vi "Inv_Mpemba1_flat potential_Host.vi"() -> ()   [LabVIEW 2019]
uses:
  <vilib>/rvi/interface/nirviMethod/nirviMethod.xnode
  <vilib>/rvi/errors/niLvFpgaMergeErrorWithErrorCode.vi
  <vilib>/rvi/interface/nirviReadWriteControl/nirviReadWriteControl.xnode
  <vilib>/rvi/interface/Simulation/niFpgaSimulationCallBeginRW.vi
  <vilib>/rvi/errors/niLvFpgaAdjustHostInterfaceError.vi
  <vilib>/Utility/file.llb/Write Delimited Spreadsheet (DBL).vi
  <vilib>/Analysis/NI_AALBase.lvlib
  <vilib>/Analysis/baseanly.llb/Mean (DBL).vi
  <vilib>/FPGAPlugInAG/Dynamic/niLvFpga_Reset_Dynamic.vi
  <vilib>/FPGAPlugInAG/Dynamic/niLvFpga_Run_Dynamic.vi
  <vilib>/rvi/interface/nirviCloseFPGA/nirviCloseFPGA.xnode
  <vilib>/rvi/interface/nirviOpenFPGA/nirviOpenFPGA.xnode
  <vilib>/FPGAPlugInAG/Dynamic/niLvFpga_ConfigureFifo_Dynamic.vi
  <vilib>/FPGAPlugInAG/Dynamic/niLvFpga_StartFifo_Dynamic.vi
  <vilib>/FPGAPlugInAG/Dynamic/niLvFpga_ReadFifo_Dynamic.vi
  <vilib>/FPGAPlugInAG/Dynamic/niLvFpga_StopFifo_Dynamic.vi
  <vilib>/FPGAPlugInAG/Dynamic/niLvFpga_Close_Dynamic.vi
panel:
  in  "Fiting Control":enum32{"Fitting Control", "Fitting Errors"}(tab)
  in  "initial\nparameters":dbl[](array[numeric])=[0.0, 9.0, 9.5, 0.0, 10.0, 8.0, 0.0]
  out "best fit parameters":sgl[](array[numeric])=[2.367998, 71.04778, 52.719345, 1362.0597, 12663.36, 64782.47]
  in  "Cal px/V":dbl=95.933 format="%#_13g"
  in  "Offset":i32=5
  out "residue":dbl
  out "Fitting in \nprogress":bool
  in  "Fit?":bool
  out "signal\n offset_X":sgl=5.0
  out "error out":errorcluster
  out "Volt":sgl[](array[numeric])
  out "Pos array":sgl[](array[numeric])
  out "smoothing error":i32
  in  "Use Cal?":bool=TRUE
  in  "Bias":sgl=0.00026
  in  "Force Wall":sgl=30.0
  in  "V_offset":sgl
  in  "Calibration":T1={"K0"=0.0, "K1"=1.0, "K2"=0.0, "K3"=0.0, "K4"=0.0, "K5"=0.0}
  in  "wait time":sgl=50.0
  in  "Calibration ON/OFF":bool=TRUE
  in  "Xmin":sgl=-1.0
  in  "Fmax":sgl=2.25
  in  "Xmax":sgl=2.0
  in  "Xoffset":sgl=0.00147
  in  "Yoffset":sgl=-0.00294
  in  "sum_offset":sgl=-0.0068
  in  "?":u16(ring) items=["No FB", "HW", "FB"]
  in  "DW":cluster{"xm":sgl, "Eb":sgl, "Tau":sgl, "dE":sgl}={"xm"=1.5, "Eb"=0.0, "Tau"=100.0, "dE"=0.0} {"dE" format="%#_3g"}
  in  "DL_Y":dbl=2.5 format="%#_13g"
  in  "TL_Y":dbl=2.5 format="%#_13g"
  in  "Stop":bool
  in  "FB time":u32=10
  in  "Triangle wave":T2={"signal offset_X"=5.0, "Scale X"=0.0, "signal offset_Y"=5.0, "Scale Y"=0.0, "Phase Shift"=30}
  in  "Elements":u32=100000
  in  "Data length":dbl=50.0
  out "Done saving":bool
  out "?":dbl=-2.0
  in  "Save Data":bool
  in  "mobX(px/V)":sgl=1.0
  in  "1/Xcali":sgl=1.0
  in  "DX":sgl=54.093
  out "Loop time":sgl=10.0 format="%.2f"
  out "Underflow":bool
  out "Fx out":sgl=5.0
  out "X":waveform(dbl)(graph)={"t0"=timestamp(0 s since 1904-01-01), "dt"=9.999999747378752e-06, "Y"=array[100000 elements]}
  out "Y":waveform(dbl)(graph)={"t0"=timestamp(0 s since 1904-01-01), "dt"=9.999999747378752e-06, "Y"=array[100000 elements]}
  out "Sum":waveform(dbl)(graph)={"t0"=timestamp(0 s since 1904-01-01), "dt"=9.999999747378752e-06, "Y"=array[100000 elements]}
  in  "Reaverage PS":bool
  out "meanX":dbl=-6.061647862558365 format="%0.5f"
  in  "Xmean":sgl
  out "PSX":dynamicdata(graph)=[{"t0"=timestamp(0 s since 1904-01-01), "dt"=1.0000000252621255, "Y"=array[50000 elements], "attributes"=variant("NI_ChannelName"=variant(string "PSD"))}]
  out "PSY":dynamicdata(graph)=[{"t0"=timestamp(0 s since 1904-01-01), "dt"=1.0000000252621255, "Y"=array[50000 elements], "attributes"=variant("NI_ChannelName"=variant(string "PSD"))}]
  out "PSsum":dynamicdata(graph)=[{"t0"=timestamp(0 s since 1904-01-01), "dt"=1.0000000252621255, "Y"=array[50000 elements], "attributes"=variant("NI_ChannelName"=variant(string "PSD"))}]
  in  "Feedback parameters":T3={"SP_QPDX"=0.0, "alpha"=0.02, "ktrap"=38.4787, "alphacounterX"=0.02135}
  in  "TW freq":dbl=1.0
  in  "Normalize signal":bool=TRUE
  out "meanY":dbl=0.25761256396234034 format="%0.5f"
  out "meanZ":dbl=0.6057344160246849 format="%0.4f"
  out "?":errorcluster
  in  "file path (dialog if empty)":path=path "C:/Users/Diffusivity/Desktop/Inverse_Mpemba_starting June16/2020 June 24/t.txt"
  # "th = 1.896"
  # "tw = 1.002"
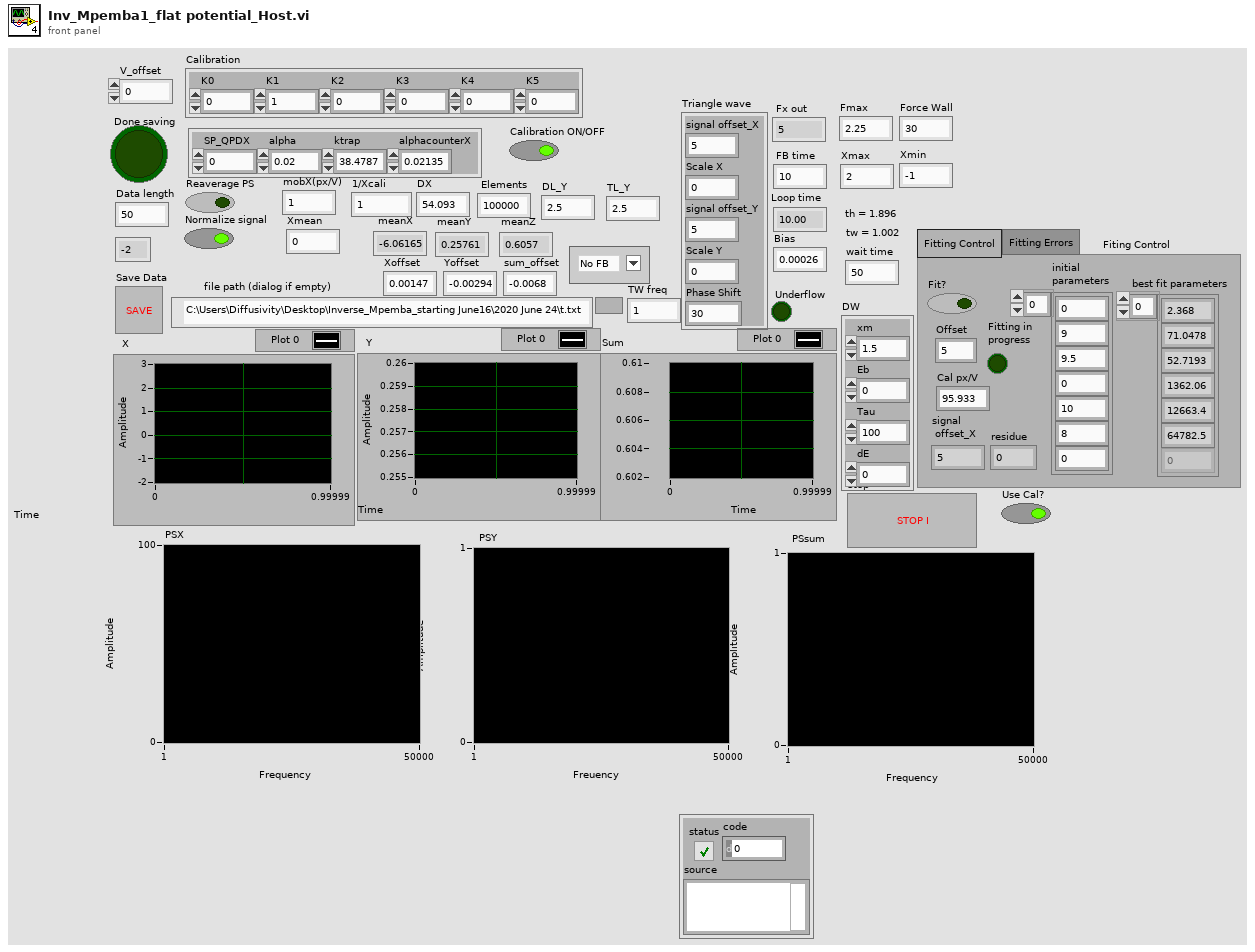
[diagram p1: front panel]
types:
  T1 = cluster{"K0":sgl, "K1":sgl, "K2":sgl, "K3":sgl, "K4":sgl, "K5":sgl}
  T2 = cluster{"signal offset_X":sgl, "Scale X":sgl, "signal offset_Y":sgl, "Scale Y":sgl, "Phase Shift":u32}
  T3 = cluster{"SP_QPDX":sgl, "alpha":sgl, "ktrap":sgl, "alphacounterX":sgl}
  T4 = cluster{"signal offset_X":sgl, "Scale X":sgl, "signal offset_Y":sgl, "Scale Y":sgl, u32}
  T5 = cluster{"[0]":sgl, "[1]":sgl, "[2]":sgl, "[3]":sgl, "[4]":sgl, "[5]":sgl}
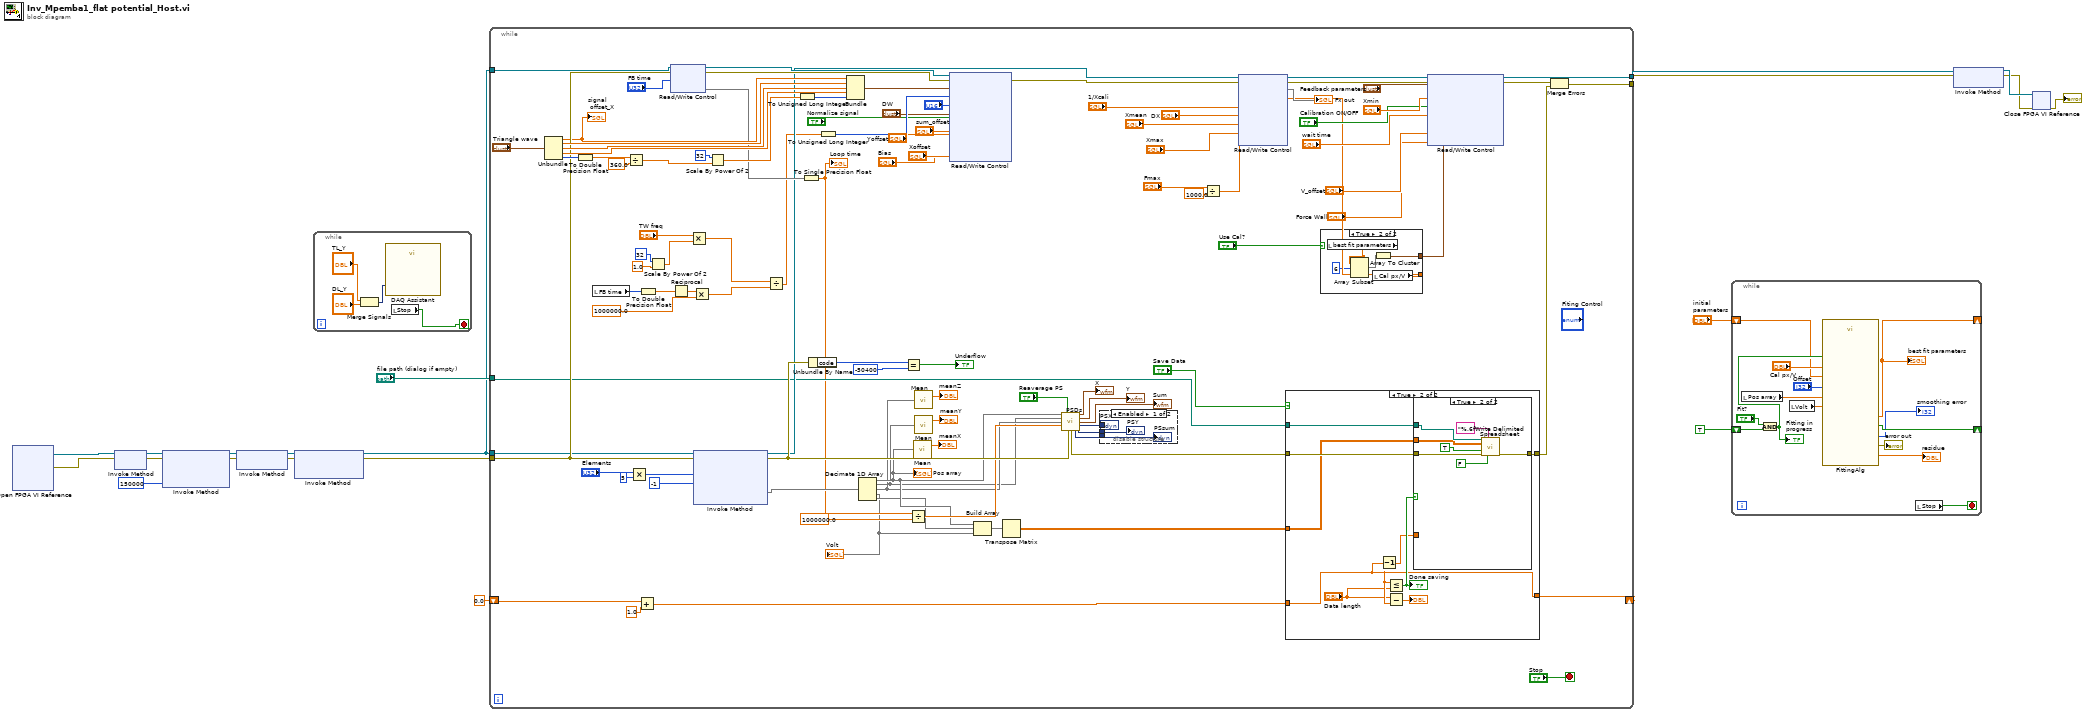
[diagram p0: block diagram]
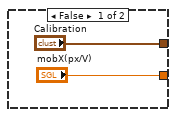
[diagram p2: hidden frame]
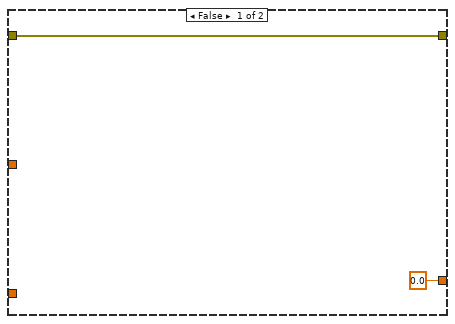
[diagram p4: hidden frame]
diagram:
  n1 = xnode "Open FPGA VI Reference"() -> ("FPGA VI Reference Out"=w4:refnum<k20>, "error out"=w3:errorcluster)  [unwired: 2 in]
  n2 = xnode "Invoke Method"("FPGA VI Reference In"=w4, "error in"=w3) -> ("FPGA VI Reference Out"=w10:refnum<k20>, "error out"=w9:errorcluster)
  n3 = xnode "Invoke Method"("FPGA VI Reference In"=w10, "error in"=w9, "Requested Depth"=u32 150000) -> ("FPGA VI Reference Out"=w15:refnum<k20>, "error out"=w14:errorcluster)  [unwired: 1 out]
  n4 = xnode "Invoke Method"("FPGA VI Reference In"=w15, "error in"=w14) -> ("FPGA VI Reference Out"=w17:refnum<k20>, "error out"=w16:errorcluster)
  n5 = xnode "Invoke Method"("FPGA VI Reference In"=w17, "error in"=w16) -> ("FPGA VI Reference Out"=w13:refnum<k20>, "error out"=w12:errorcluster)  [unwired: 1 in]
  n6 = while {
    stop <- w21 stop-if-true
    n7 = Merge Signals("TL_Y", "DL_Y") -> (w24:dynamicdata)
    n8 = call "DAQ Assistant"("data"=w24) -> ()  [unwired: 17 in, 2 out]
    n9 = local read "Stop"() -> (w21:bool)
  }
  n10 = while {
    tunnel: w13 -> [w101]
    tunnel: w12 -> [w102]
    tunnel: "file path (dialog if empty)" -> [w69]
    tunnel: [w94] -> w19
    tunnel: [w107] -> w18
    tunnel: w13 -> [w88]
    shift-right: [w98] -> _
    shift-left: 0.0 -> [w97]
    stop <- "Stop" stop-if-true
    n11 = Unbundle("Triangle wave") -> ("signal offset_X"=w91:sgl, "Scale X"=w111:sgl, "signal offset_Y"=w110:sgl, "Scale Y"=w109:sgl, "Phase Shift"=w112:u32)
    "signal\n offset_X" <- w91
    n12 = To Double Precision Float(number=w112) -> (double precision float=w118:dbl)
    n13 = local read "FB time"() -> (w59:u32)
    n14 = Divide(x=w118, y=360.0) -> (x/y=w116:dbl)
    n15 = Multiply(x="Elements", y=u32 5) -> (x*y=w103:u32)
    n16 = Add(x=w97, y=1.0) -> (x+y=w99:dbl)
    n17 = To Double Precision Float(number=w59) -> (double precision float=w60:dbl)
    n18 = Scale By Power Of 2(n=i16 32, x=1.0) -> (x*2^n=w64:dbl)
    n19 = xnode "Read/Write Control"("FPGA VI Reference In"=w101, "error in"=w102, "FB Time"="FB time") -> ("FPGA VI Reference Out"=w123:refnum<k20>, "error out"=w89:errorcluster, "FB Time"=w87)
    n20 = Reciprocal(x=w60) -> (1/x=w61:dbl)
    n21 = Multiply(x="TW freq", y=w64) -> (x*y=w57:dbl)
    n22 = Multiply(x=w61, y=1000000.0) -> (x*y=w56:dbl)
    n23 = xnode "Invoke Method"("FPGA VI Reference In"=w88, "error in"=w102, "Number of Elements"=w103, "Timeout (ms)"=-1) -> ("FPGA VI Reference Out"=w71:refnum<k20>, "error out"=w85:errorcluster, "Data"=w80:void[])  [unwired: 1 out]
    n24 = Scale By Power Of 2(n=i16 32, x=w116) -> (x*2^n=w114:dbl)
    n25 = Divide(x=w57, y=w56) -> (x/y=w55:dbl)
    n26 = To Unsigned Long Integer(number=w114) -> (unsigned 32bit integer=w108:u32)
    n27 = To Single Precision Float(number=w87) -> (single precision float=w66:sgl)
    "Loop time" <- w66
    n28 = Unbundle By Name(w85) -> ("code"=w106:i32)
    n29 = To Unsigned Long Integer(number=w55) -> (unsigned 32bit integer=w54:u32)
    n30 = Bundle("signal offset_X"=w91, "Scale X"=w111, "signal offset_Y"=w110, "Scale Y"=w109, w108) -> (w67:T4)  [unwired: 1 in]
    n31 = Decimate 1D Array(w80) -> (w48:void[], w33:void[], w46:void[], w44:void[], w47:void[])
    "Pos array" <- w48
    "Volt" <- w44
    n32 = Equal?(x=w106, y=-50400) -> (x = y?=→"Underflow":bool)
    n33 = Divide(x=w66, y=sgl 1000000.0) -> (x/y=w49:sgl)
    n34 = call-poly <vilib>:"Mean.vi"("X"=w48) -> ("mean"=→"meanX":dbl)  [unwired: 1 out]
    n35 = call-poly <vilib>:"Mean.vi"("X"=w46) -> ("mean"=→"meanZ":dbl)  [unwired: 1 out]
    n36 = call-poly <vilib>:"Mean.vi"("X"=w33) -> ("mean"=→"meanY":dbl)  [unwired: 1 out]
    n37 = xnode "Read/Write Control"("FPGA VI Reference In"=w123, "error in"=w89, "Triangle wave"=w67, "Frequency"=w54, "Enum"="?", "DW"="DW", "Normalize signal"="Normalize signal", "sum_offset"="sum_offset", "Yoffset"="Yoffset", "Xoffset"="Xoffset", "Bias"="Bias") -> ("error out"=w70:errorcluster)  [unwired: 1 out]
    n38 = Build Array(w48, w47, w44) -> (w92:void[])
    n39 = Transpose Matrix(1:w92) -> (0:w121:dbl[][])
    n40 = call "PSDs.vi"("X"=w48, "averaging done"="Reaverage PS", "Y"=w33, "sum"=w46, "dt"=w49, "error in (no error)"=w85) -> ("X"=→"X":waveform(dbl), "Y"=→"Y":waveform(dbl), "Sum"=→"Sum":waveform(dbl), "PSDX"=w76:dynamicdata, "error out"=w84:errorcluster, "PSDsum"=w74:dynamicdata, "PSDY"=w75:dynamicdata)  [unwired: 3 in]
    n41 = disable-structure shown="Enabled" {
      disable-tunnel: w76 -> [w135 _]
      disable-tunnel: w75 -> [w134 _]
      disable-tunnel: w74 -> [w133 _]
      frame Enabled {
        "PSX" <- w135
        "PSY" <- w134
        "PSsum" <- w133
      }
      frame Disabled {
      }
    }
    n42 = Divide(x="Fmax", y=sgl 1000.0) -> (x/y=w36:sgl)
    n43 = case shown="True" "Save Data" {
      tunnel: w121 -> [_ w141]
      tunnel: w69 -> [_ w146]
      tunnel: w84 -> [w137 w145]
      tunnel: [w137 w144] -> w120
      tunnel: w99 -> [_ w140]
      tunnel: [0.0 w140] -> w98
      frame False {
      }
      frame True {
        n44 = Decrement(x=w140) -> (x-1=w139:dbl)
        n45 = Less Or Equal?(x=w140, y="Data length") -> (x <= y?=w143:bool)
        "Done saving" <- w143
        n46 = Subtract(x="Data length", y=w140) -> (x-y=→"?":dbl)
        n47 = case shown="True" w143 {
          tunnel: w141 -> [_ w148]
          tunnel: w146 -> [_ w149]
          tunnel: w145 -> [w147 w152]
          tunnel: [w147 w151] -> w144
          tunnel: w139 -> [_ _]
          frame False {
          }
          frame True {
            n48 = call-poly <vilib>:"Write Delimited Spreadsheet.vi"("file path (dialog if empty)"=w149, "format (%.3f)"="%.6f", "2D data"=w148, "append to file? (new file:F)"=TRUE, "error in (no error)"=w152, "transpose? (no:F)"=FALSE) -> ("error out"=w151:errorcluster)  [unwired: 8 in, 1 out]
          }
        }
      }
    }
    n49 = case shown="True" "Use Cal?" {
      tunnel: ["Calibration" w132] -> w27
      tunnel: ["mobX(px/V)" w128] -> w26
      frame False {
      }
      frame True {
        n50 = local read "best fit parameters"() -> (w130:sgl[])
        n51 = Array Subset(array=w130, length=6) -> (w129:sgl[])  [unwired: 1 in]
        n52 = local read "Cal px/V"() -> (w128:dbl)
        n53 = Array To Cluster(array=w129) -> (cluster=w132:T5)
      }
    }
    n54 = xnode "Read/Write Control"("FPGA VI Reference In"=w71, "error in"=w70, "MobX(px/V)"=w26, "1/Xcali"="1/Xcali", "DX"="DX", "Xmean"="Xmean", "Xmax"="Xmax", "Fmax"=w36) -> ("FPGA VI Reference Out"=w96:refnum<k20>, "error out"=w95:errorcluster, "Fx out"=→"Fx out")
    n55 = xnode "Read/Write Control"("FPGA VI Reference In"=w96, "error in"=w95, "Feedback parameters"="Feedback parameters", "Xmin"="Xmin", "Calibration ON/OFF"="Calibration ON/OFF", "wait time"="wait time", "Calibration"=w27, "V_offset"="V_offset", "Force"="Force Wall") -> ("FPGA VI Reference Out"=w94:refnum<k20>, "error out"=w93:errorcluster)
    n56 = Merge Errors(w93, w120) -> (w107:errorcluster)
  }
  n57 = while {
    shift-right: [w168] -> _
    shift-left: "initial\nparameters" -> [w155]
    shift-right: [w159] -> _
    shift-left: TRUE -> [w163]
    stop <- w160 stop-if-true
    n58 = local read "Pos array"() -> (w167:sgl[])
    n59 = And(x="Fit?", y=w163) -> (x .and. y?=w161:bool)
    "Fitting in \nprogress" <- w161
    n60 = local read "Volt"() -> (w166:sgl[])
    n61 = call "FittingAlg.vi"("Pos"=w167, "Cal px/V"="Cal px/V", "initial parameters"=w155, "Volt"=w166, "Boolean in"=w161, "Offset"="Offset") -> ("error"=→"smoothing error":i32, "best fit parameters"=w168:dbl[], "Boolean out"=w159:bool, "residue"=→"residue":dbl, "error out"=→"error out":errorcluster)  [unwired: 5 in]
    "best fit parameters" <- w168
    n62 = local read "Stop"() -> (w160:bool)
  }
  n63 = xnode "Invoke Method"("FPGA VI Reference In"=w19, "error in"=w18) -> ("FPGA VI Reference Out"=w8:refnum<k20>, "error out"=w7:errorcluster)
  n64 = xnode "Close FPGA VI Reference"("FPGA VI Reference In"=w8, "error in"=w7) -> ("error out"=→"?":errorcluster)
